vi "Shoot Initialize.vi"(9 "refnum name":string="Shoot Talon", 10 "Shoot Master":u8, 11 "Shoot Slave":u8) -> ()   [LabVIEW 2019]
uses:
  <vilib>/Rock Robotics/WPI/ThirdParty/Phoenix-LabVIEW/Motor Controller/Controls/CTRE_Phoenix_MotorControl_NeutralMode.ctl
  .Team Code/Contants.vi
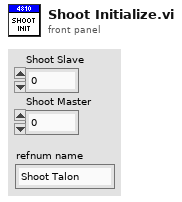
[diagram p1: front panel]
types:
  T1 = typedef "CTRE_Phoenix_MotorControl_NeutralMode.ctl" = enum8{"EEPROMSetting", "Override to Coast", "Override to Brake"}
  T2 = enum16{"FollowerType_PercentOutput", "FollowerType_AuxOutput1"}
  T3 = typedef "WPI_MotorControlDeviceRef.ctl" = cluster{"DeviceStatus":errorcluster, "Type":T4, "PWM":cluster{"PWM Channel":T5, "DeadBand":T6}, "CAN":cluster{"Device Number":u8, "SetOutput VI Ref":variant, "GetOutput VI Ref":variant, "Enable VI Ref":variant, "Disable VI Ref":variant, "Data":variant}, "Invert":bool, "DIO PWM":cluster{"PWM \"Enable\" Channel":T5, "DIOChannel":T7, "PWM Rate":dbl}}
  T4 = typedef "WPI_MotorControlType.ctl" = enum16{"PWM", "CAN", "DIO PWM"}
  T5 = typedef "FPGA_DIOPWMChannel.ctl" = enum8{"PWM 0", "PWM 1", "PWM 2", "PWM 3", "PWM 4", "PWM 5", "PWM 6", "PWM 7", "PWM 8", "PWM 9", "PWM MXP 0", "PWM MXP 1", "PWM MXP 2", "PWM MXP 3", "PWM MXP 4", "PWM MXP 5", "PWM MXP 6", "PWM MXP 7", "PWM MXP 8", "PWM MXP 9", "Invalid"}
  T6 = typedef "WPI_PWMDeadband.ctl" = cluster{"Name":string, "maxPositivePwm":i32, "minPositivePwm":i32, "centerPwm":i32, "maxNegativePwm":i32, "minNegativePwm":i32, "angularRange":u16}
  T7 = typedef "FPGA_DIOChannel.ctl" = enum8{"DIO 0", "DIO 1", "DIO 2", "DIO 3", "DIO 4", "DIO 5", "DIO 6", "DIO 7", "DIO 8", "DIO 9", "DIO MXP 0", "DIO MXP 1", "DIO MXP 2", "DIO MXP 3", "DIO MXP 4", "DIO MXP 5", "DIO MXP 6", "DIO MXP 7", "DIO MXP 8", "DIO MXP 9", "DIO MXP 10", "DIO MXP 11", "DIO MXP 12", "DIO MXP 13", "DIO MXP 14", "DIO MXP 15", "SPI Port CS1", "SPI Port CS2", "SPI Port CS3", "SPI Port MISO", "SPI Port MOSI", "Invalid"}
  T8 = cluster{"Cruise Velocity":i32, "Acceleration":i32}
  T9 = cluster{"P":dbl, "I":dbl, "D":dbl, "F":dbl, "I Zone":dbl}
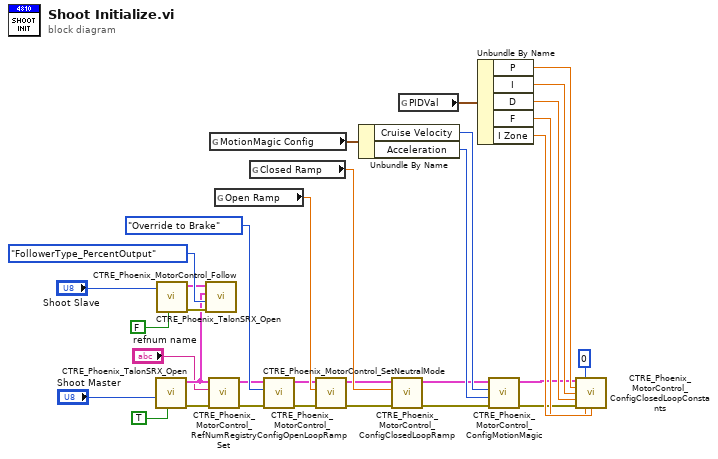
[diagram p0: block diagram]
diagram:
  n1 = call <vilib>:"CTRE_Phoenix_TalonSRX_Open.vi"("Invert"=TRUE, "Device Number"="Shoot Master") -> ("error out"=w16:errorcluster, "CAN Talon SRX Ref"=w6:T3)  [unwired: 8 in]
  n2 = call <vilib>:"CTRE_Phoenix_TalonSRX_Open.vi"("Invert"=FALSE, "Device Number"="Shoot Slave") -> ("error out"=w17:errorcluster, "CAN Talon SRX Ref"=w5:T3)  [unwired: 8 in]
  n3 = call <vilib>:"CTRE_Phoenix_MotorControl_Follow.vi"("error in (no error)"=w17, "FollowerType"=T2."FollowerType_PercentOutput", "Master Controller to Follow"=w6, "PhoenixMotorControlDevRef"=w5) -> ()  [unwired: 6 in, 2 out]
  n4 = call <vilib>:"CTRE_Phoenix_MotorControl_RefNumRegistrySet.vi"("error in (no error)"=w16, "refnum name"="refnum name", "PhoenixMotorControlDevRef"=w6) -> ("error out"=w15:errorcluster, "PhoenixMotorControlDevRef"=w9:T3)  [unwired: 7 in]
  n5 = global read "Contants.vi" "MotionMagic Config"() -> (w22:T8)
  n6 = global read "Contants.vi" "Open Ramp"() -> (w32:dbl)
  n7 = global read "Contants.vi" "Closed Ramp"() -> (w31:dbl)
  n8 = call <vilib>:"CTRE_Phoenix_MotorControl_SetNeutralMode.vi"("error in (no error)"=w15, "Motor Control Neutral Mode"=CTRE_Phoenix_MotorControl_NeutralMode."Override to Brake", "PhoenixMotorControlDevRef"=w9) -> ("error out"=w14:errorcluster, "PhoenixMotorControlDevRef"=w11:T3)  [unwired: 7 in]
  n9 = call <vilib>:"CTRE_Phoenix_MotorControl_ConfigOpenLoopRamp.vi"("error in (no error)"=w14, "secondsFromNeutralToFull"=w32, "PhoenixMotorControlDevRef"=w11) -> ("error out"=w12:errorcluster, "PhoenixMotorControlDevRef"=w13:T3)  [unwired: 7 in]
  n10 = Unbundle By Name(w22) -> ("Cruise Velocity"=w23:i32, "Acceleration"=w24:i32)
  n11 = call <vilib>:"CTRE_Phoenix_MotorControl_ConfigClosedLoopRamp.vi"("error in (no error)"=w12, "secondsFromNeutralToFull"=w31, "PhoenixMotorControlDevRef"=w13) -> ("error out"=w21:errorcluster, "PhoenixMotorControlDevRef"=w18:T3)  [unwired: 7 in]
  n12 = global read "Contants.vi" "PIDVal"() -> (w25:T9)
  n13 = Unbundle By Name(w25) -> ("P"=w26:dbl, "I"=w27:dbl, "D"=w28:dbl, "F"=w29:dbl, "I Zone"=w30:dbl)
  n14 = call <vilib>:"CTRE_Phoenix_MotorControl_ConfigMotionMagic.vi"("error in (no error)"=w21, "Acceleration"=w24, "Cruise Velocity"=w23, "PhoenixMotorControlDevRef"=w18) -> ("error out"=w20:errorcluster, "PhoenixMotorControlDevRef"=w19:T3)  [unwired: 6 in]
  n15 = call <vilib>:"CTRE_Phoenix_MotorControl_ConfigClosedLoopConstants.vi"("PhoenixMotorControlDevRef"=w19, "slotIdx"=0, "P"=w26, "I"=w27, "D"=w28, "error in (no error)"=w20, "F"=w29, "I Zone"=w30) -> ()  [unwired: 6 in, 2 out]
